vi "ACal-Find Multiband Edges.vi"(0 "Freq":dbl[](array[numeric]), 5 "Mag":dbl[](array[numeric]), 7 "Fmin":dbl, 9 "Fmax":dbl, 11 "Max Range":dbl) -> (4 "Fstart":dbl[](array[numeric]), 8 "Istart":i32[](array[numeric]), 15 "Mags":dbl[](array[numeric]))   [LabVIEW 2020]
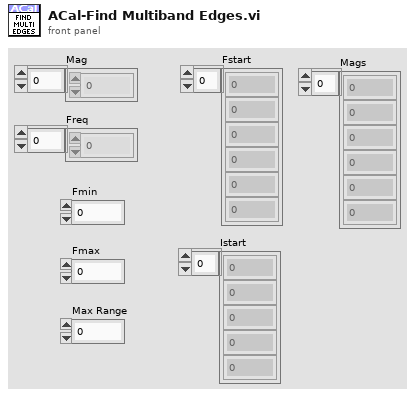
[diagram p1: front panel]
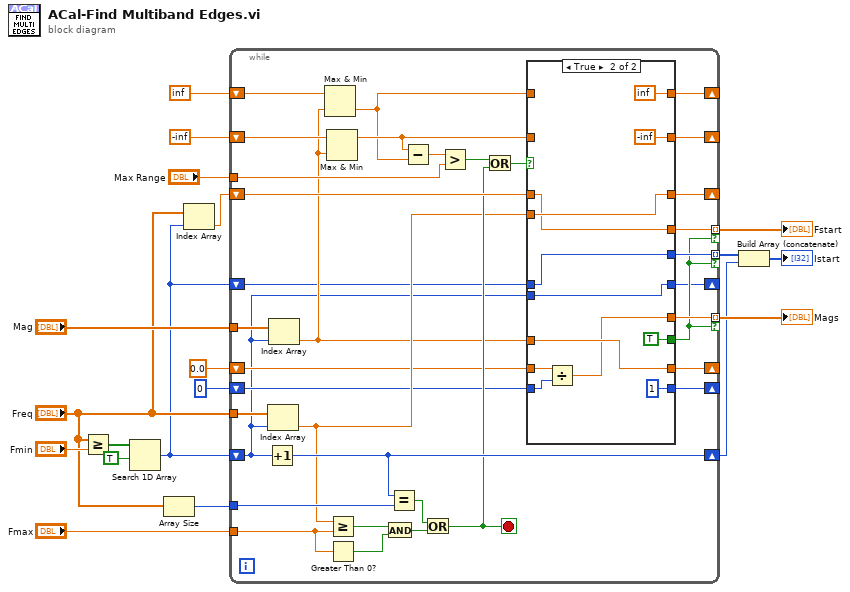
[diagram p0: block diagram]
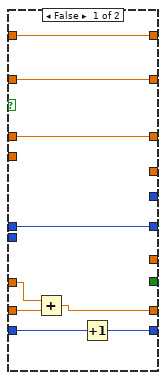
[diagram p2: hidden frame]
diagram:
  n1 = Greater Or Equal?(x="Freq", y="Fmin") -> (x >= y?=w18:bool[])
  n2 = Search 1D Array(1D array=w18, element=TRUE) -> (index of element=w1:i32)  [unwired: 1 in]
  n3 = Array Size(array="Freq") -> (size(s)=w12:i32)
  n4 = Index Array(array="Freq", index=w1) -> (element=w9:dbl)
  n5 = while {
    tunnel: "Freq" -> [w54]
    tunnel: "Mag" -> [w46]
    shift-right: [w38] -> _
    shift-left: inf -> [w45]
    shift-right: [w40] -> _
    shift-left: -inf -> [w44]
    shift-right: [w48] -> w3
    shift-left: w1 -> [w20]
    tunnel: "Fmax" -> [w51]
    tunnel: w12 -> [w47]
    tunnel: "Max Range" -> [w42]
    shift-right: [w32] -> _
    shift-left: w9 -> [w36]
    tunnel: [w31] -> w8 mode=indexing if=w23
    tunnel: [w30] -> w7 mode=indexing if=w23
    shift-right: [w25] -> _
    shift-left: 0.0 -> [w29]
    shift-right: [w26] -> _
    shift-left: 0 -> [w27]
    tunnel: [w24] -> w5 mode=indexing if=w23
    shift-right: [w21] -> _
    shift-left: w1 -> [w22]
    stop <- w34 stop-if-true
    n6 = Increment(x=w20) -> (x+1=w48:i32)
    n7 = Index Array(array=w54, index=w20) -> (element=w33:dbl)
    n8 = Index Array(array=w46, index=w20) -> (element=w28:dbl)
    n9 = Max & Min(x=w45, y=w28) -> (min(x,y)=w37:dbl)  [unwired: 1 out]
    n10 = Max & Min(x=w44, y=w28) -> (max(x,y)=w39:dbl)  [unwired: 1 out]
    n11 = Greater Or Equal?(x=w33, y=w51) -> (x >= y?=w53:bool)
    n12 = Greater Than 0?(x=w51) -> (x > 0?=w52:bool)
    n13 = And(x=w53, y=w52) -> (x .and. y?=w50:bool)
    n14 = Equal?(x=w48, y=w47) -> (x = y?=w49:bool)
    n15 = Subtract(x=w39, y=w37) -> (x-y=w43:dbl)
    n16 = Or(x=w49, y=w50) -> (x .or. y?=w34:bool)
    n17 = Greater?(x=w43, y=w42) -> (0:w41:bool)
    n18 = Or(x=w41, y=w34) -> (x .or. y?=w35:bool)
    n19 = case shown="True" w35 {
      tunnel: [w63 -inf] -> w40
      tunnel: w39 -> [w63 _]
      tunnel: [w62 inf] -> w38
      tunnel: w37 -> [w62 _]
      tunnel: w36 -> [w61 w72]
      tunnel: w33 -> [_ w73]
      tunnel: [w61 w73] -> w32
      tunnel: [_ w72] -> w31
      tunnel: [_ w65] -> w30
      tunnel: [_ TRUE] -> w23
      tunnel: w29 -> [w58 w68]
      tunnel: w28 -> [w57 w69]
      tunnel: w27 -> [w60 w67]
      tunnel: [w59 1] -> w26
      tunnel: [w56 w69] -> w25
      tunnel: [_ w66] -> w24
      tunnel: w22 -> [w55 w65]
      tunnel: [w55 w64] -> w21
      tunnel: w20 -> [_ w64]
      frame False {
        n20 = Add(x=w57, y=w58) -> (x+y=w56:dbl)
        n21 = Increment(x=w60) -> (x+1=w59:i32)
      }
      frame True {
        n22 = Divide(x=w68, y=w67) -> (x/y=w66:dbl)
      }
    }
  }
  "Fstart" <- w8
  "Mags" <- w5
  n23 = Build Array (concatenate)(w7, w3) -> (→"Istart":i32[])
